vi "History Get Current Version.vi"(8 "error in (no error)":errorcluster, 11 "Connection Refnum":T2) -> (0 "error out":errorcluster, 2 "Current Version Record":T1, 3 "Connection Refnum":T2)   [LabVIEW 2011]
uses:
  Summitek EXT/ODBC/SQL Controls/Connection Refnum.ctl
  History Record.ctl
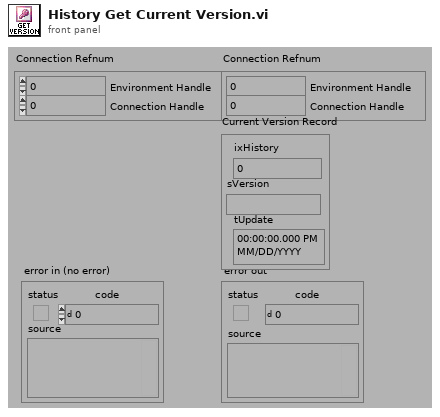
[diagram p1: front panel]
types:
  T1 = typedef "History Record.ctl" = cluster{"ixHistory":i32, "sVersion":string, "tUpdate":timestamp}
  T2 = typedef "Connection Refnum.ctl" = cluster{"Environment Handle":i32, "Connection Handle":i32}
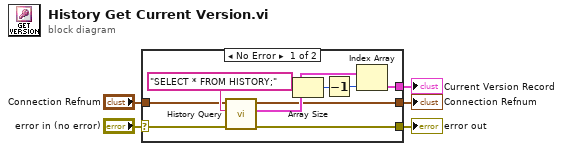
[diagram p0: block diagram]
diagram:
  n1 = case shown="No Error" "error in (no error)" {
    selector: "error in (no error)" -> [w6 w16]
    tunnel: [w10 _] -> w5
    tunnel: [w9 w15] -> w4
    tunnel: [w8 w16] -> w3
    tunnel: "Connection Refnum" -> [w7 w15]
    frame No Error {
      n2 = call "History Query.vi"("error in (no error)"=w6, "Query"="SELECT * FROM HISTORY;", "Connection Refnum"=w7) -> ("error out"=w8:errorcluster, "History Record"=w13:T1[], "Connection Refnum"=w9:T2)  [unwired: 6 out]
      n3 = Array Size(array=w13) -> (size(s)=w12:i32)
      n4 = Decrement(x=w12) -> (x-1=w11:i32)
      n5 = Index Array(array=w13, index=w11) -> (element=w10:T1)
    }
    frame Error {
    }
  }
  "error out" <- w3
  "Connection Refnum" <- w4
  "Current Version Record" <- w5
